vi "Calculate R assign_v2.vi"(6 "deform array":dbl[](array[numeric])=[1.0, 1.0, 1.0, 0.0, 0.0, 0.0, 0.0, 0.0, 0.0], 8 "AssignPoint":dbl[](array[numeric]), 9 "EyeCenter":dbl[](array[numeric]), 10 "r_max":dbl, 11 "r_eye":dbl) -> (1 "Tassign":dbl[](array[numeric]), 3 "r_assign":dbl)   [LabVIEW 2010]
doc: "This VI calulates the assigned radius based on the formula:\nAssignPointRadius = min(EyeRadius - norm([ EyeCenter(1)-AssignPoint(1), EyeCenter(2)-AssignPoint(2) ],2),AssignPointRadiusMax)\n\nIf calculated AssignPointRadius is negative, namely the assign point is outside of the workspace, Rcalc would be 0 and Tcalc would be the starting point of the baseline trajectory."
uses:
  <vilib>/Analysis/NI_AALPro.lvlib
  <vilib>/Analysis/_algsub.llb/Real Vector Norm.vi
  <vilib>/Analysis/_algsub.llb/Vector Norm Type.ctl
  <vilib>/Analysis/NI_AALBase.lvlib
  <vilib>/Analysis/baseanly.llb/A x Vector.vi
  <vilib>/Analysis/Matrix/NI_Matrix.lvlib
  <vilib>/Analysis/Matrix/Numeric/Conversions/Array To Matrix - RA2.vi
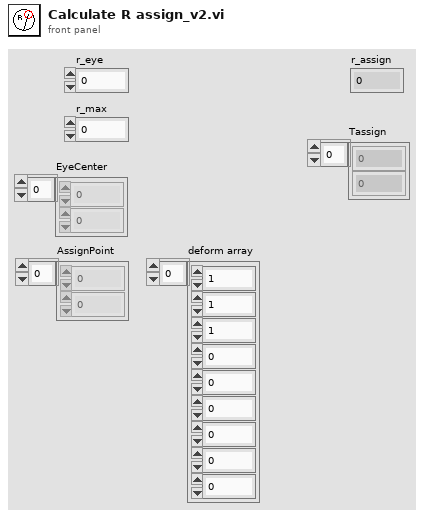
[diagram p1: front panel]
types:
  T1 = typedef "NI_AALPro.lvlib/Vector Norm Type.ctl" = u16
  T2 = typedef "NI_Matrix.lvlib/RealMatrix.ctl" = dbl[][]
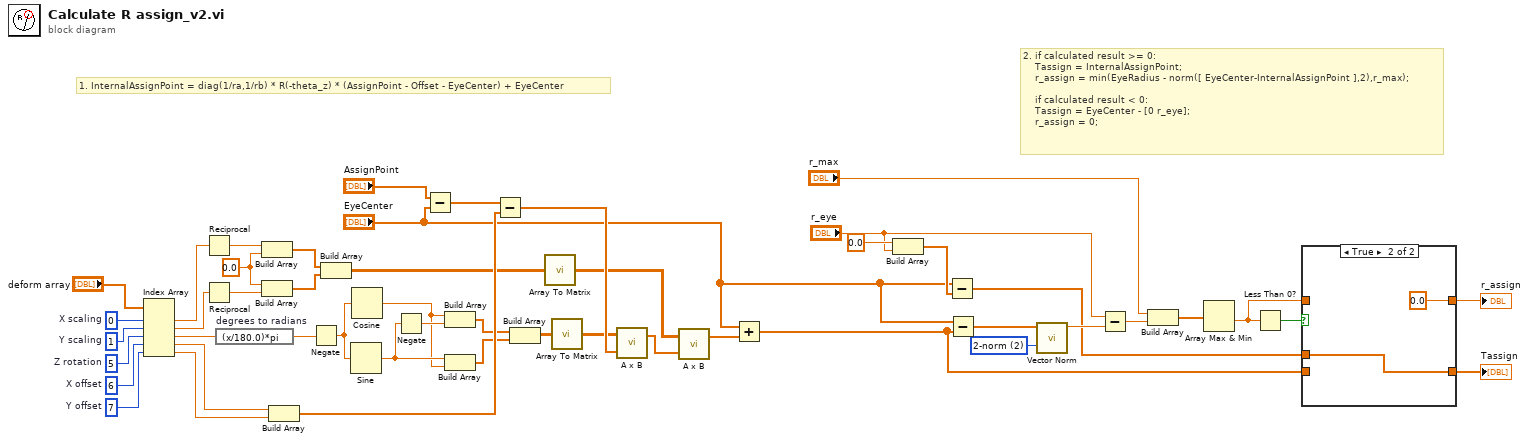
[diagram p0: block diagram]
diagram:
  w25 = 0.0 ("element")
  w30 = 7  # Y offset
  w31 = 6  # X offset
  w32 = 5  # Z rotation
  w33 = 1  # Y scaling
  w34 = 0  # X scaling
  w48 = T1 2 items=["1-norm"=1, "2-norm"=2, "Inf-norm"=3, "-Inf-norm"=4, "User Defined"=5] ("norm type")
  # "1. InternalAssignPoint = diag(1/ra,1/rb) * R(-theta_z) * (AssignPoint - Offset - EyeCenter) + EyeCenter"
  # "2. if calculated result >= 0:\n    Tassign = InternalAssignPoint;\n    r_assign = min(EyeRadius - norm([ EyeCenter-InternalAssignPoint ],2),r_max);\n\n    if calculated result < 0:\n    Tassign = EyeCenter - [0 r_eye];\n    r_assign = 0;"
  n1 = Index Array(array="deform array", index #1=w34, index #2=w33, index #3=w32, index #4=w31, index #5=w30) -> (element #1=w29:dbl, element #2=w28:dbl, element #3=w17:dbl, element #4=w22:dbl, element #5=w21:dbl)
  n2 = Reciprocal(x=w29) -> (1/x=w26:dbl)
  n3 = Reciprocal(x=w28) -> (1/x=w27:dbl)
  n4 = expression code="(x/180.0)*pi" "degrees to radians"(w17) -> (w16:dbl)
  n5 = Build Array(w26, w25) -> (w24:dbl[])
  n6 = Build Array(w25, w27) -> (w23:dbl[])
  n7 = Build Array(w22, w21) -> (w19:dbl[])
  n8 = Negate(x=w16) -> (-x=w15:dbl)
  n9 = Build Array(w24, w23) -> (w5:dbl[][])
  n10 = Sine(x=w15) -> (sin(x)=w13:dbl)
  n11 = Cosine(x=w15) -> (cos(x)=w12:dbl)
  n12 = Negate(x=w13) -> (-x=w14:dbl)
  n13 = Subtract(x="AssignPoint", y="EyeCenter") -> (x-y=w18:dbl[])
  n14 = Build Array(w12, w14) -> (w11:dbl[])
  n15 = Build Array(w13, w12) -> (w10:dbl[])
  n16 = Subtract(x=w18, y=w19) -> (x-y=w8:dbl[])
  n17 = Build Array(w11, w10) -> (w9:dbl[][])
  n18 = call-poly <vilib>:"Array To Matrix.vi"("Real 2D Array"=w5) -> ("Real Matrix"=w4:T2)
  n19 = call-poly <vilib>:"Array To Matrix.vi"("Real 2D Array"=w9) -> ("Real Matrix"=w7:T2)
  n20 = call-poly <vilib>:"A x B.vi"("Vector"=w8, "A"=w7) -> ("A x Vector"=w6:dbl[])  [unwired: 1 out]
  n21 = call-poly <vilib>:"A x B.vi"("Vector"=w6, "A"=w4) -> ("A x Vector"=w3:dbl[])  [unwired: 1 out]
  n22 = Add(x="EyeCenter", y=w3) -> (x+y=w2:dbl[])
  n23 = Build Array(0.0 ("element"), "r_eye") -> (w39:dbl[])
  n24 = Subtract(x="EyeCenter", y=w39) -> (x-y=w38:dbl[])
  n25 = Subtract(x="EyeCenter", y=w2) -> (x-y=w49:dbl[])
  n26 = call-poly <vilib>:"Vector Norm.vi"("norm type"=w48, "Input Vector"=w49) -> ("norm"=w47:dbl)  [unwired: 8 in, 1 out]
  n27 = Subtract(x="r_eye", y=w47) -> (x-y=w45:dbl)
  n28 = Build Array("r_max", w45) -> (w44:dbl[])
  n29 = Array Max & Min(array=w44) -> (min value=w41:dbl)  [unwired: 3 out]
  n30 = Less Than 0?(x=w41) -> (x < 0?=w43:bool)
  n31 = case shown="True" w43 {
    tunnel: [w51 0.0] -> w42
    tunnel: w41 -> [w51 _]
    tunnel: w2 -> [w50 _]
    tunnel: [w50 w52] -> w40
    tunnel: w38 -> [_ w52]
    frame False {
    }
    frame True {
    }
  }
  "r_assign" <- w42
  "Tassign" <- w40
